vi "gaz protection.vi"() -> ()   [LabVIEW 2016]
doc: "Read one the value of one analog channel from a LINX device."
uses:
  <vilib>/MakerHub/LINX/Public/Peripherals/Analog/Analog Read 1 Chan.vi
  <vilib>/MakerHub/LINX/Public/Peripherals/Digital/Digital Write 1 Chan.vi
  <vilib>/MakerHub/LINX/Public/Peripherals/Analog/Analog Read N Chans.vi
  <vilib>/MakerHub/LINX/Public/Peripherals/Digital/Digital Write N Chans.vi
  <vilib>/MakerHub/LINX/Private/Local IO/LinxAnalogRead.vi
  <vilib>/MakerHub/LINX/Public/Utilities/Check Channel.vi
  <vilib>/MakerHub/LINX/Private/Local IO/LinxDigitalWrite.vi
  <vilib>/MakerHub/LINX/Public/Utilities/Open Serial.vi
  <vilib>/MakerHub/LINX/Private/Utilties/Generate Error.vi
  <vilib>/MakerHub/LINX/Public/Sensors/Motion/Servo/Servo Open One Channel.vi
  <vilib>/MakerHub/LINX/Public/Sensors/Motion/Servo/Servo Set Pulse Width One Channel.vi
  <vilib>/MakerHub/LINX/LMH-LINX.lvlib
  <vilib>/MakerHub/LINX/Public/Sensors/Motion/Servo/Servo.lvlib
panel:
  out "?":bool
  out "?":bool
  out "?":bool
  out "?":bool
  in  "Servo Channel":u8
  in  "capteur feu":u8
  in  "Led":u8
  in  "ventillateur":u8
  in  "buzzer":u8
  in  "Stop Button":bool
  out "Analog Data":dbl(graph)
  out "Loop Rate (Hz)":u32
  in  "Serial Port":refnum<visa-resource-name>
  # "LINX Device Settings"
  # "Analog Value"
  # "Actuators"
  # "Pins"
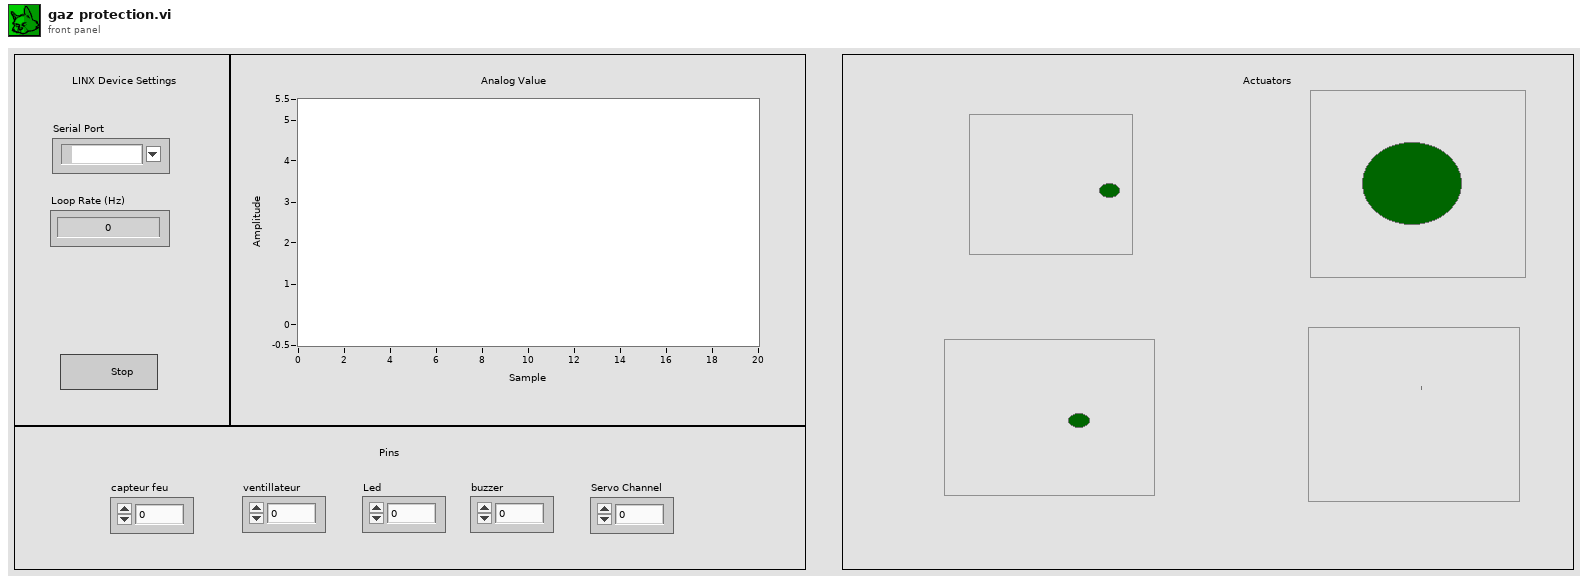
[diagram p1: front panel]
types:
  T1 = typedef "LMH-LINX.lvlib/LINX Ref.ctl" = cluster{"IO":T2, "Interface":T3, "LINX Device Config":T4}
  T2 = typedef "LMH-LINX.lvlib/Platform.ctl" = enum16{"Remote", "Local"}
  T3 = typedef "LMH-LINX.lvlib/Interface.ctl" = enum16{"Serial", "TCP"}
  T4 = typedef "LMH-LINX.lvlib/Device.lvlib/LINX Device Config.ctl" = cluster{"Interface":T3, "COM Port":refnum<visa-resource-name>, "TCP Configuration":T5, "Device Family":u8, "Device ID":u8, "Device Name":string, "TCP Ref":refnum<k5>, "Channels":T6}
  T5 = typedef "LMH-LINX.lvlib/Device.lvlib/TCP Config.ctl" = cluster{"IP Address":string, "Port":u16}
  T6 = typedef "LMH-LINX.lvlib/Channels.ctl" = cluster{"DI":u8[], "DO":u8[], "AI":u8[], "AO":u8[], "PWM":u8[], "QE":u8[], "UART":u8[], "I2C 2":u8[], "SPI":u8[], "CAN":u8[], "Servo":u8[], "AI Ref (V)":dbl, "AI Resolution (Bits)":u8, "AO Ref (V)":dbl, "AO Resolution (Bits)":u8}
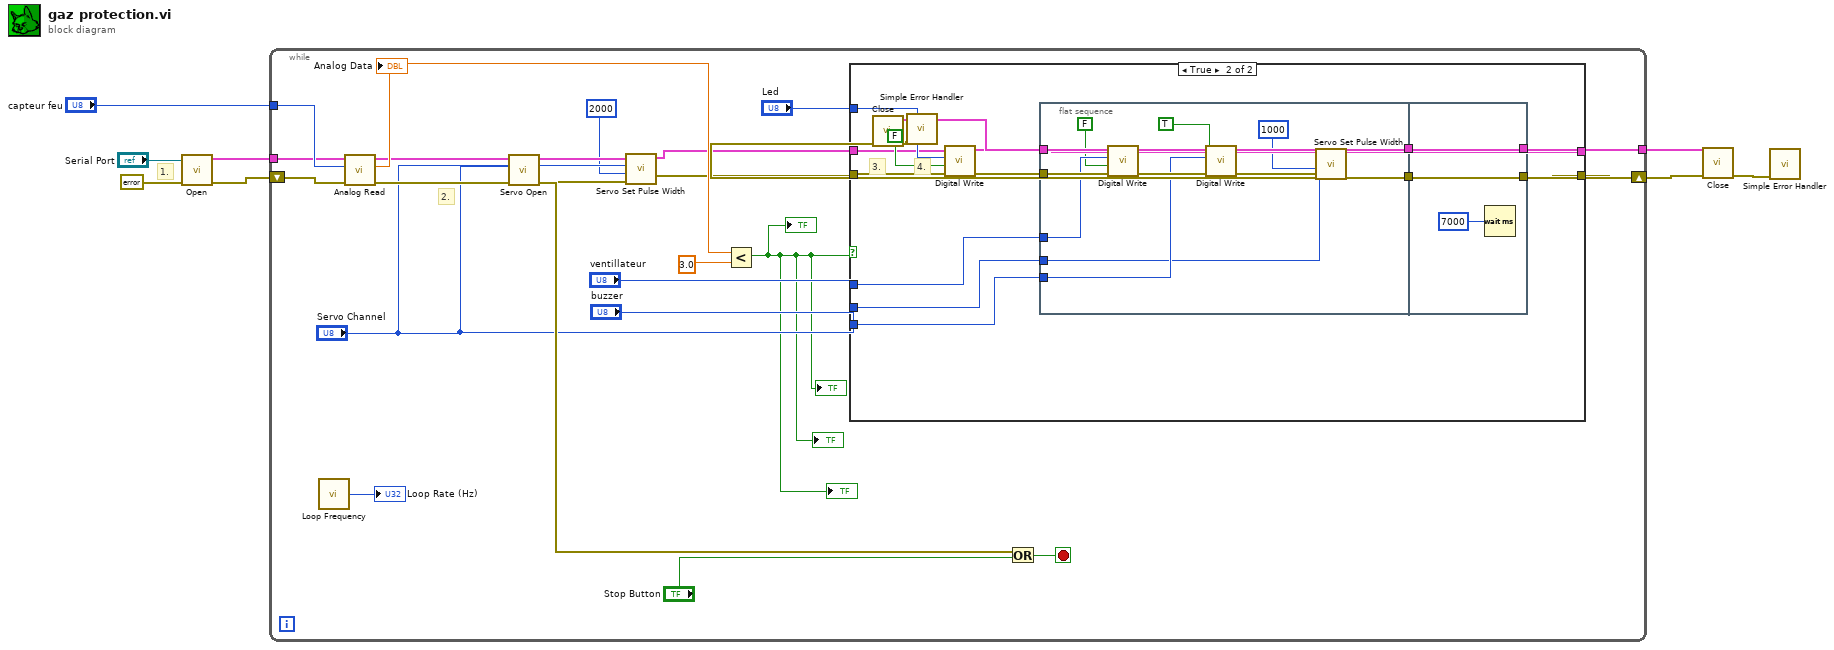
[diagram p0: block diagram]
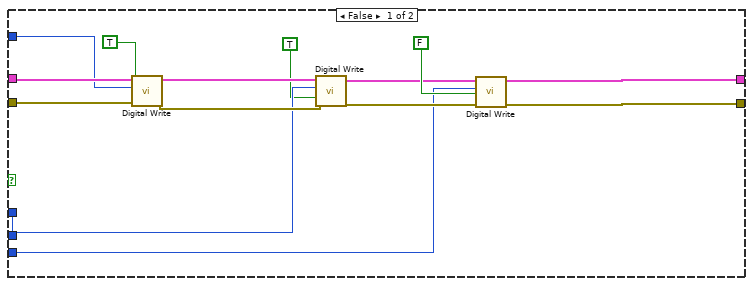
[diagram p2: hidden frame]
diagram:
  # "4."
  # "3."
  # "1."
  n1 = call-poly <vilib>:"Open.vi"("Error In"=errorcluster {"status"=FALSE, "code"=0, "source"=""}, "Serial Port"="Serial Port") -> ("Error Out"=w8:errorcluster, "LINX Resource"=w9:T1)  [unwired: 7 in, 1 out]
  n2 = while {
    tunnel: w9 -> [w20]
    shift-right: [w21] -> w2
    shift-left: w8 -> [w19]
    tunnel: "capteur feu" -> [w28]
    tunnel: [w22] -> w3
    stop <- w31 stop-if-true
    # "2."
    n3 = call <vilib>:"Loop Frequency.vi"() -> ("Loop Rate (Hz)"=→"Loop Rate (Hz)":u32)
    n4 = call-poly <vilib>:"Analog Read.vi"("Error In"=w19, "Analog Channel"=w28, "LINX Resource"=w20) -> ("Error Out"=w17:errorcluster, "Voltage"=w27:dbl, "LINX Resource"=w18:T1)  [unwired: 5 in, 1 out]
    "Analog Data" <- w27
    n5 = call-poly <vilib>:"Servo Open.vi"("Error In"=w17, "Servo Channel"="Servo Channel", "LINX Resource"=w18) -> ("Error Out"=w15:errorcluster, "LINX Resource"=w16:T1)  [unwired: 7 in]
    n6 = call-poly <vilib>:"Servo Set Pulse Width.vi"("Error In"=w15, "Pulse Width (uS)"=u16 2000, "Servo Channel"="Servo Channel", "LINX Resource"=w16) -> ("Error Out"=w13:errorcluster, "LINX Resource"=w14:T1)  [unwired: 6 in]
    n7 = Less?(x=w27, y=3.0) -> (x < y?=w10:bool)
    "?" <- w10
    "?" <- w10
    "?" <- w10
    "?" <- w10
    n8 = case shown="True" w10 {
      tunnel: "Led" -> [w43 w58]
      tunnel: w14 -> [w45 w56]
      tunnel: w13 -> [w44 w55]
      tunnel: "ventillateur" -> [w39 w52]
      tunnel: "buzzer" -> [w34 w51]
      tunnel: [w33 w50] -> w22
      tunnel: [w32 w49] -> w21
      tunnel: "Servo Channel" -> [_ w46]
      frame False {
        n9 = call-poly <vilib>:"Digital Write.vi"("Error In"=w44, "Output Value"=TRUE, "DO Channel"=w43, "LINX Resource"=w45) -> ("Error Out"=w40:errorcluster, "LINX Resource"=w41:T1)  [unwired: 6 in]
        n10 = call-poly <vilib>:"Digital Write.vi"("Error In"=w40, "Output Value"=TRUE, "DO Channel"=w39, "LINX Resource"=w41) -> ("Error Out"=w35:errorcluster, "LINX Resource"=w36:T1)  [unwired: 6 in]
        n11 = call-poly <vilib>:"Digital Write.vi"("Error In"=w35, "Output Value"=FALSE, "DO Channel"=w34, "LINX Resource"=w36) -> ("Error Out"=w32:errorcluster, "LINX Resource"=w33:T1)  [unwired: 6 in]
      }
      frame True {
        n12 = call-poly <vilib>:"Digital Write.vi"("Error In"=w55, "Output Value"=FALSE, "DO Channel"=w58, "LINX Resource"=w56) -> ("Error Out"=w53:errorcluster, "LINX Resource"=w54:T1)  [unwired: 6 in]
        n13 = flat-sequence {
          tunnel: w54 -> [w72]
          tunnel: w53 -> [w71]
          tunnel: w52 -> [w70]
          tunnel: w51 -> [w66]
          tunnel: [w60] -> w48
          tunnel: [w59] -> w47
          tunnel: w46 -> [w64]
          tunnel: [w74] -> w49
          tunnel: [w75] -> w50
          tunnel: w48 -> [w75]
          tunnel: w47 -> [w74]
          frame #0 {
            n14 = call-poly <vilib>:"Digital Write.vi"("Error In"=w71, "Output Value"=FALSE, "DO Channel"=w70, "LINX Resource"=w72) -> ("Error Out"=w67:errorcluster, "LINX Resource"=w68:T1)  [unwired: 6 in]
            n15 = call-poly <vilib>:"Digital Write.vi"("Error In"=w67, "Output Value"=TRUE, "DO Channel"=w66, "LINX Resource"=w68) -> ("Error Out"=w61:errorcluster, "LINX Resource"=w62:T1)  [unwired: 6 in]
            n16 = call-poly <vilib>:"Servo Set Pulse Width.vi"("Error In"=w61, "Pulse Width (uS)"=u16 1000, "Servo Channel"=w64, "LINX Resource"=w62) -> ("Error Out"=w59:errorcluster, "LINX Resource"=w60:T1)  [unwired: 6 in]
          }
          frame #1 {
            n17 = Wait (ms)(milliseconds to wait=u32 7000) -> ()  [unwired: 1 out]
          }
        }
      }
    }
    n18 = Or(x=w17, y="Stop Button") -> (x .or. y?=w31:bool)
  }
  n19 = call <vilib>:"Close.vi"("Error In"=w2, "LINX Resource"=w3) -> ("Error Out"=w6:errorcluster)  [unwired: 9 in]
  n20 = call <vilib>:"Simple Error Handler.vi"("error in (no error)"=w6) -> ()  [unwired: 4 in, 5 out]
  n21 = call <vilib>:"Close.vi"("Error In"=w2, "LINX Resource"=w3) -> ("Error Out"=w1:errorcluster)  [unwired: 9 in]
  n22 = call <vilib>:"Simple Error Handler.vi"("error in (no error)"=w1) -> ()  [unwired: 4 in, 5 out]
